vi "Check ADC status.vi"(5 "ADC Status":T1, 11 "error in (no error)":errorcluster) -> (15 "error out":errorcluster)   [LabVIEW 2019]
uses:
  <instrlib>/niMmWave/ni3610 and ni3630/controls/public/ADC Status.ctl
  <instrlib>/niMmWave/ni3610 and ni3630/ni3610_and_ni3630_Driver_Lib.lvlib
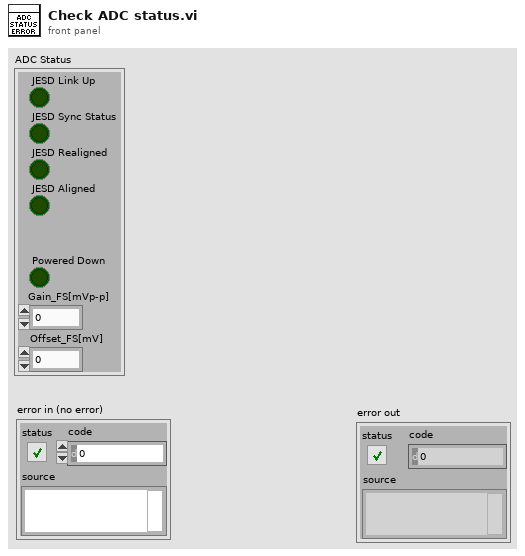
[diagram p1: front panel]
types:
  T1 = typedef "ni3610_and_ni3630_Driver_Lib.lvlib/ADC Status.ctl" = cluster{"JESD Link Up":bool, "JESD Sync Status":bool, "JESD Realigned":bool, "JESD Aligned":bool, "Powered Down":bool, "Gain_FS[mVp-p]":dbl, "Offset_FS[mV]":dbl}
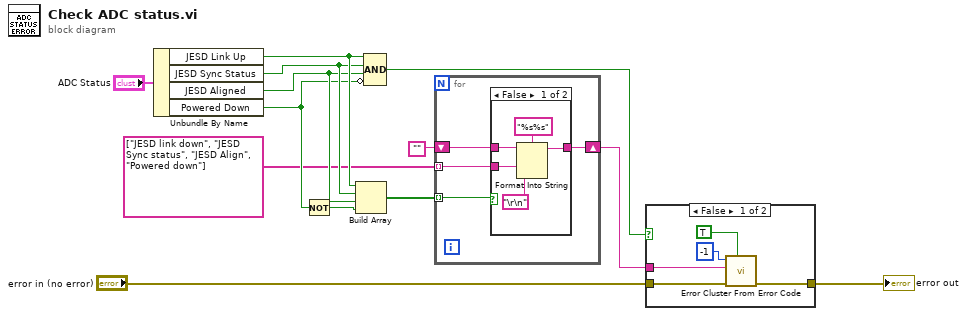
[diagram p0: block diagram]
diagram:
  n1 = Unbundle By Name("ADC Status") -> ("JESD Link Up"=w9:bool, "JESD Sync Status"=w8:bool, "JESD Aligned"=w7:bool, "Powered Down"=w6:bool)
  n2 = Not(x=w6) -> (.not. x?=w5:bool)
  n3 = Build Array(w9, w8, w7, w5) -> (w4:bool[])
  n4 = Compound Arithmetic op=AND(w9, w8, w7, invert w6) -> (w10:bool)
  n5 = for {
    tunnel: w4 -> [w17] mode=indexing
    shift-right: [w15] -> w2
    shift-left: "" -> [w16]
    tunnel: string[] ["JESD link down", "JESD Sync status", "JESD Align", "Powered down"] -> [w14] mode=indexing
    n6 = case shown="False" w17 {
      tunnel: w16 -> [w22 w23]
      tunnel: [w19 w23] -> w15
      tunnel: w14 -> [w18 _]
      frame False {
        n7 = Format Into String(format string="%s%s", initial string=w22, w18, "\r\n") -> (resulting string=w19:string)  [unwired: 1 in, 1 out]
      }
      frame True {
      }
    }
  }
  n8 = case shown="False" w10 {
    tunnel: "error in (no error)" -> [w28 w29]
    tunnel: [w27 w29] -> w11
    tunnel: w2 -> [w25 _]
    frame False {
      n9 = call <vilib>:"Error Cluster From Error Code.vi"("show call chain? (False)"=TRUE, "error in (no error)"=w28, "error message (\"\")"=w25, "error code (0)"=-1) -> ("error out"=w27:errorcluster)  [unwired: 5 in]
    }
    frame True {
    }
  }
  "error out" <- w11
